vi "Acquire.vi"(8 "error in (no error)":errorcluster, 11 "Strain in":refnum<class "Strain.lvclass">) -> (0 "error out":errorcluster, 3 "Strain out":refnum<class "Strain.lvclass">)   [LabVIEW 2013, in "Strain.lvlib" / "Strain.lvclass"]
uses:
  Strain.lvclass
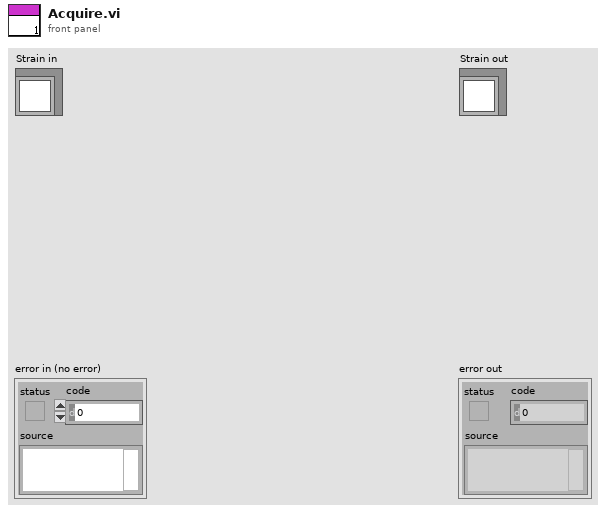
[diagram p1: front panel]
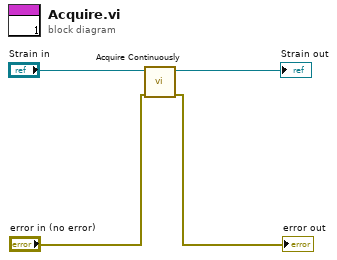
[diagram p0: block diagram]
diagram:
  n1 = call-dynamic "Acquire Continuously.vi"("error in (no error)"="error in (no error)", "Strain in"="Strain in") -> ("error out"=→"error out":errorcluster, "Strain out"=→"Strain out":refnum<class "Strain.lvclass">)  [unwired: 8 in]
